vi "Show Detail.vi"(6 "mnu file Path 2":path, 7 "mnu file Path 1":path, 8 "error in (no error)":errorcluster, 9 "Palettes Different?":bool, 10 "Palette data array 2":T5(array[cluster]) {"view format" items=["Icons", "Text", "Icons and Text"]}, 11 "Palette data array 1":T5(array[cluster]) {"view format" items=["Icons", "Text", "Icons and Text"]}) -> (0 "error out":errorcluster)   [LabVIEW 2017]
uses:
  <vilib>/Palette API/Palette Menu/Public Type Define/View Format.ctl
  <vilib>/Palette API/Palette Menu/Public Type Define/Items.ctl
  <vilib>/Palette API/Palette Menu/Public Type Define/Item.ctl
  <vilib>/Palette API/Palette Menu/Public Type Define/Synchronize Info.ctl
  <vilib>/Palette API/Palette Menu/Palette Menu.lvlib
panel:
  out "Picture 2":picture
  in  "mnu file 2":string
  out "Picture 1":picture
  in  "mnu file 1":string
  in  "Palette information":string(tree)
  in  "View Format":T1 items=["Icons", "Text", "Icons and Text"]
  in  "stop":bool
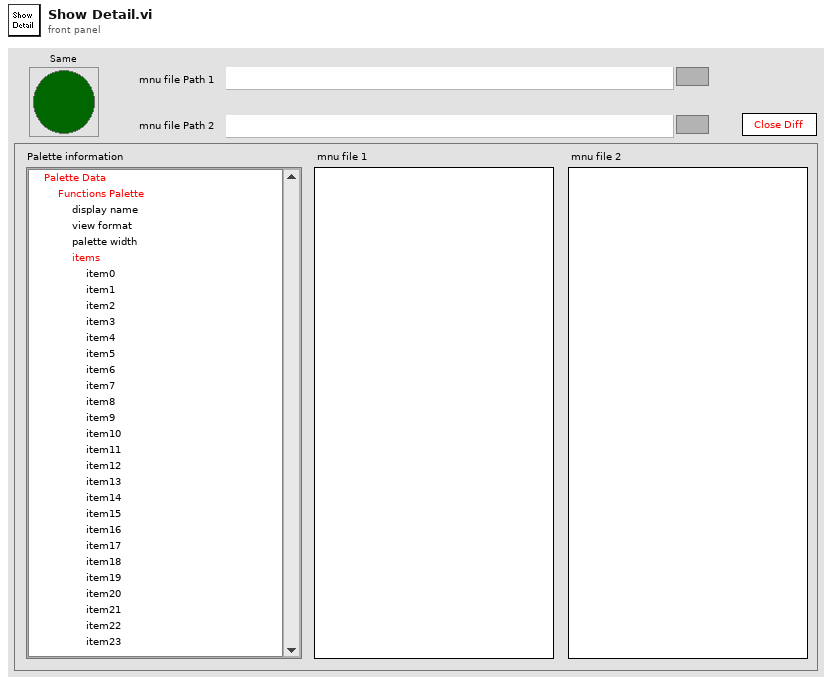
[diagram p1: front panel]
types:
  T1 = typedef "Palette Menu.lvlib/View Format.ctl" = u16
  T2 = typedef "Palette Menu.lvlib/Items.ctl" = T3[]
  T3 = typedef "Palette Menu.lvlib/Item.ctl" = cluster{"item path":path, "library path (.lvlib)":path, "use default lvlib palette":bool, "short name":string, "place VI contents":bool, "hide synchronized item":bool, "reserve spot for synch item":bool, "configure when placing VI contents":bool}
  T4 = typedef "Palette Menu.lvlib/Synchronize Info.ctl" = cluster{"synchronize with directory":bool, "synchronize directory path":path}
  T5 = cluster{"display name":string, "view format":T1, "palette width":i16, "items":T2, "256 color icon":picture, "B&W color icon":picture, "help information":cluster{"help tag":string, "help file path":path}, "palette description":string, "synchronize information":T4}[]
  T6 = enum32{"Invalid", "Standard", "Closed", "Hidden", "Minimized", "Maximized"}
  T7 = cluster{"display name":string, "view format":T1, "palette width":i16, "items":T2, "256 color icon":picture, "B&W color icon":picture, "help information":cluster{"help tag":string, "help file path":path}, "palette description":string, "synchronize information":T4}
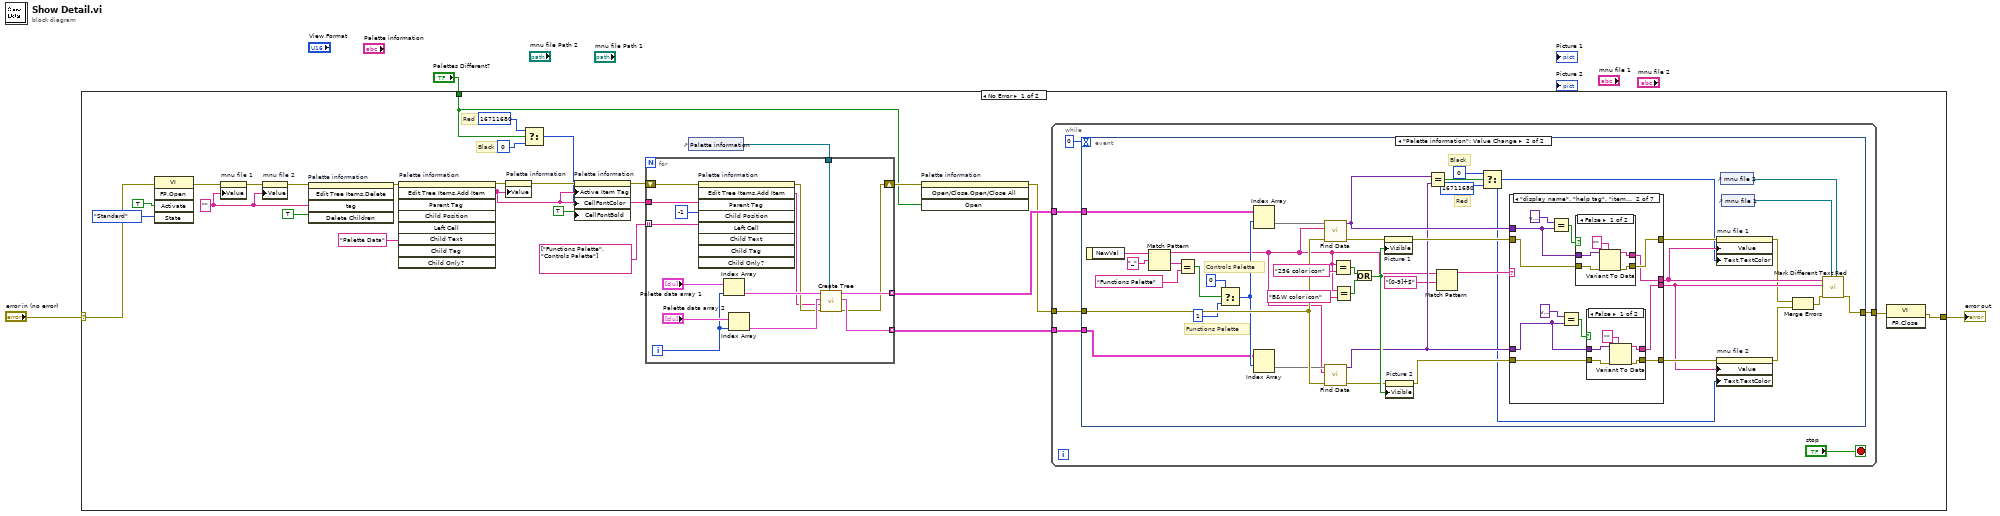
[diagram p0: block diagram]
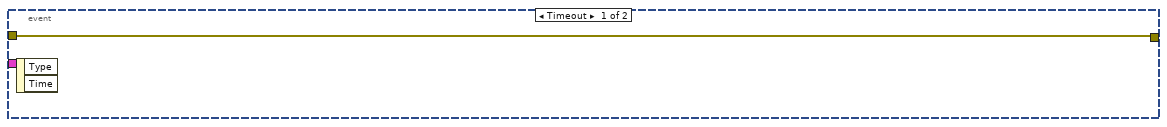
[diagram p2: hidden frame]
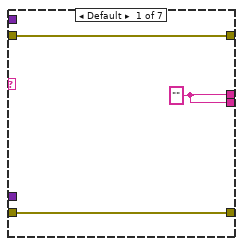
[diagram p3: hidden frame]
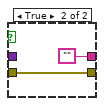
[diagram p4: hidden frame]
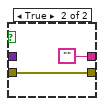
[diagram p5: hidden frame]
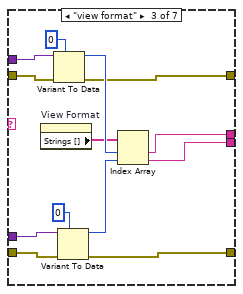
[diagram p6: hidden frame]
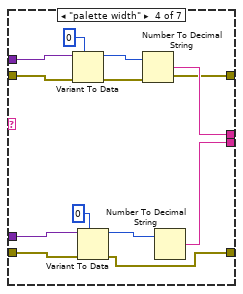
[diagram p7: hidden frame]
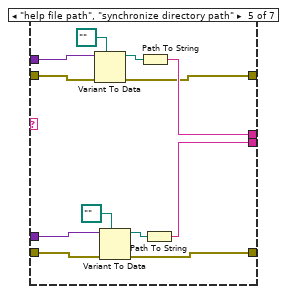
[diagram p8: hidden frame]
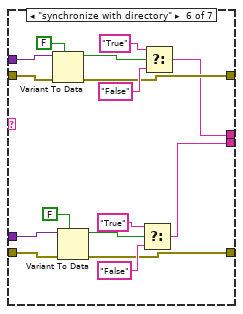
[diagram p9: hidden frame]
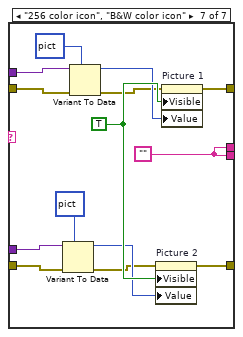
[diagram p10: hidden frame]
diagram:
  n1 = case shown="No Error" "error in (no error)" {
    selector: "error in (no error)" -> [w30 w190]
    tunnel: [w27 w190] -> w2
    tunnel: "Palettes Different?" -> [w4 _]
    frame No Error {
      w19 = "" ("Tag")
      # "Red"
      # "Black"
      n2 = invoke class="VI" method="FP.Open"(error in=w30, "Activate"=TRUE ("Activate?"), "State"=T6."Standard") -> (error out=w20:errorcluster)  [unwired: 2 in, 4 out]
      n3 = property on="mnu file 1" class="Str"(error in=w20, "Value"=w19) -> (error out=w22:errorcluster)  [unwired: 1 in, 1 out]
      n4 = property on="mnu file 2" class="Str"(error in=w22, "Value"=w19) -> (error out=w21:errorcluster)  [unwired: 1 in, 1 out]
      n5 = invoke on="Palette information" class="Tree (strict)" method="Edit Tree Items.Delete"(error in=w21, "tag"=w19, "Delete Children"=TRUE ("Delete Children?")) -> (error out=w25:errorcluster)  [unwired: 2 in, 4 out]
      n6 = invoke on="Palette information" class="Tree (strict)" method="Edit Tree Items.Add Item"(error in=w25, "Left Cell"="Palette Data" ("Left Cell String")) -> (error out=w18:errorcluster, "Edit Tree Items:Add Item"=w10:string)  [unwired: 7 in, 7 out]
      n7 = property on="Palette information" class="Tree (strict)"(error in=w18, "Value"=w10) -> (error out=w13:errorcluster)  [unwired: 1 in, 1 out]
      n8 = Select(t=u32 16711680, s=w4, f=u32 0 ("t")) -> (s? t:f=w9:u32)
      n9 = property on="Palette information" class="Tree (strict)"(error in=w13, "Active Item Tag"=w10, "CellFontColor"=w9, "CellFontBold"=TRUE ("Active Cell:Cell Font:Bold")) -> (error out=w7:errorcluster)  [unwired: 1 in, 1 out]
      n10 = control-ref of="Palette information"() -> (w16:refnum<vi>)
      n11 = for {
        tunnel: w10 -> [w44]
        tunnel: string[] ["Functions Palette", "Controls Palette"] ("Palette type") -> [w37] mode=indexing
        tunnel: w16 -> [w38]
        tunnel: [w35] -> w15 mode=indexing
        shift-right: [w31] -> w6
        shift-left: w7 -> [w34]
        tunnel: [w33] -> w14 mode=indexing
        i -> [w40]
        n12 = invoke on="Palette information" class="Tree (strict)" method="Edit Tree Items.Add Item"(error in=w34, "Parent Tag"=w44, "Child Position"=-1, "Left Cell"=w37) -> (error out=w36:errorcluster, "Edit Tree Items:Add Item"=w32:string)  [unwired: 5 in, 7 out]
        n13 = Index Array(array="Palette data array 1", index=w40) -> (element=w42:T7)
        n14 = Index Array(array="Palette data array 2", index=w40) -> (element=w39:T7)
        n15 = call "Create Tree.vi"("Tree Refnum"=w38, "error in"=w36, "Parent Tag"=w32, "palette data 2"=w39, "palette data 1"=w42) -> ("error out"=w31:errorcluster, "data array 2"=w33:cluster{"Label":string, "Data":variant}[], "data array 1"=w35:cluster{"Label":string, "Data":variant}[])  [unwired: 4 out]
      }
      n16 = invoke on="Palette information" class="Tree (strict)" method="Open/Close.Open/Close All"(error in=w6, "Open"=w4) -> (error out=w5:errorcluster)  [unwired: 2 in, 3 out]
      n17 = while {
        tunnel: w5 -> [w49]
        tunnel: [w48] -> w23
        tunnel: w15 -> [w47]
        tunnel: w14 -> [w46]
        stop <- "stop" stop-if-true
        n18 = event shown="[1] \"Palette information\": Value Change" {
          selector: _ -> [_ _]
          dyn-events: _ -> [_ _]
          timeout: 0 -> [_ _]
          tunnel: w49 -> [w52 w82]
          tunnel: [w52 w53] -> w48
          tunnel: w47 -> [_ w76]
          tunnel: w46 -> [_ w69]
          event Timeout {
            n19 = event-data() -> ()  [unwired: 3 out]
          }
          event "Palette information": Value Change {
            # "Controls Palette"
            # "Functions Palette"
            # "Red"
            # "Black"
            n20 = event-data() -> ("NewVal"=w73:string)  [unwired: 1 out]
            n21 = Match Pattern(string=w73, regular expression="_" ("search string")) -> (before substring=w63:string, after substring=w72:string)  [unwired: 3 out]
            n22 = Equal?(x=w72, y="Functions Palette") -> (x = y?=w70:bool)
            n23 = Select(t=0 ("y"), s=w70, f=1 ("y")) -> (s? t:f=w75:i32)
            n24 = Index Array(array=w76, index (row)=w75) -> (element=w67:cluster{"Label":string, "Data":variant}[])  [unwired: 1 in]
            n25 = Index Array(array=w69, index (row)=w75) -> (element=w66:cluster{"Label":string, "Data":variant}[])  [unwired: 1 in]
            n26 = call "Find Data.vi"("error in (no error)"=w82, "Label"=w63, "data array 1"=w67) -> ("error out"=w83:errorcluster, "Value"=w68:variant)  [unwired: 7 out]
            n27 = call "Find Data.vi"("error in (no error)"=w82, "Label"=w63, "data array 1"=w66) -> ("error out"=w81:errorcluster, "Value"=w65:variant)  [unwired: 1 in, 6 out]
            n28 = Equal?(x=w63, y="256 color icon") -> (x = y?=w91:bool)
            n29 = Equal?(x=w63, y="B&W color icon") -> (x = y?=w90:bool)
            n30 = Or(x=w91, y=w90) -> (x .or. y?=w89:bool)
            n31 = property on="Picture 1" class="Pict"(error in=w83, "Visible"=w89) -> (error out=w88:errorcluster)  [unwired: 1 in, 1 out]
            n32 = property on="Picture 2" class="Pict"(error in=w81, "Visible"=w89) -> (error out=w87:errorcluster)  [unwired: 1 in, 1 out]
            n33 = Equal?(x=w68, y=w65) -> (x = y?=w86:bool)
            n34 = Match Pattern(string=w63, regular expression="[0-9]+$") -> (before substring=w62:string)  [unwired: 4 out]
            n35 = Select(t=u32 0, s=w86, f=u32 16711680) -> (s? t:f=w58:u32)
            n36 = case shown="\"display name\", \"help tag\", \"item\", \"palette description\"" w62 {
              tunnel: w87 -> [w94 w99 w127 w141 w153 w165 w181]
              tunnel: w88 -> [w95 w108 w129 w142 w154 w166 w183]
              tunnel: w68 -> [_ w103 w130 w143 w155 w167 w184]
              tunnel: w65 -> [_ w100 w128 w140 w152 w164 w182]
              tunnel: [w96 w106 w126 w139 w149 w162 w178] -> w59
              tunnel: [w95 w107 w125 w138 w148 w163 w176] -> w80
              tunnel: [w96 w97 w124 w137 w151 w160 w178] -> w57
              tunnel: [w94 w98 w123 w136 w150 w161 w177] -> w79
              frame Default {
                w96 = ""
              }
              frame "display name", "help tag", "item", "palette description" {
                n37 = Equal?(x=variant ("y"), y=w103) -> (x = y?=w104:bool)
                n38 = Equal?(x=variant ("y"), y=w100) -> (x = y?=w101:bool)
                n39 = case shown="False" w104 {
                  tunnel: w108 -> [w119 w121]
                  tunnel: [w118 w121] -> w107
                  tunnel: [w117 ""] -> w106
                  tunnel: w103 -> [w116 _]
                  frame False {
                    n40 = Variant To Data(error in=w119, type="", Variant=w116) -> (data=w117:string, error out=w118:errorcluster)
                  }
                  frame True {
                  }
                }
                n41 = case shown="False" w101 {
                  tunnel: w99 -> [w112 w114]
                  tunnel: [w111 w114] -> w98
                  tunnel: [w110 ""] -> w97
                  tunnel: w100 -> [w109 _]
                  frame False {
                    n42 = Variant To Data(error in=w112, type="", Variant=w109) -> (data=w110:string, error out=w111:errorcluster)
                  }
                  frame True {
                  }
                }
              }
              frame "view format" {
                n43 = property on="View Format" class="Ring (strict)"() -> ("Strings []"=w133:string[])  [unwired: 2 in, 2 out]
                n44 = Variant To Data(error in=w129, type=0, Variant=w130) -> (data=w134:i32, error out=w125:errorcluster)
                n45 = Variant To Data(error in=w127, type=0, Variant=w128) -> (data=w131:i32, error out=w123:errorcluster)
                n46 = Index Array(array=w133, index #1=w134, index #2=w131) -> (element #1=w126:string, element #2=w124:string)
              }
              frame "palette width" {
                n47 = Variant To Data(error in=w142, type=0, Variant=w143) -> (data=w147:i32, error out=w138:errorcluster)
                n48 = Variant To Data(error in=w141, type=0, Variant=w140) -> (data=w146:i32, error out=w136:errorcluster)
                n49 = Number To Decimal String(number=w147) -> (decimal integer string=w139:string)  [unwired: 1 out]
                n50 = Number To Decimal String(number=w146) -> (decimal integer string=w137:string)  [unwired: 1 out]
              }
              frame "help file path", "synchronize directory path" {
                n51 = Variant To Data(error in=w154, type=path "", Variant=w155) -> (data=w157:path, error out=w148:errorcluster)
                n52 = Variant To Data(error in=w153, type=path "", Variant=w152) -> (data=w156:path, error out=w150:errorcluster)
                n53 = Path To String(path=w157) -> (string=w149:string)
                n54 = Path To String(path=w156) -> (string=w151:string)
              }
              frame "synchronize with directory" {
                n55 = Variant To Data(error in=w166, type=FALSE, Variant=w167) -> (data=w168:bool, error out=w163:errorcluster)
                n56 = Variant To Data(error in=w165, type=FALSE, Variant=w164) -> (data=w174:bool, error out=w161:errorcluster)
                n57 = Select(t="True", s=w174, f="False") -> (s? t:f=w160:string)
                n58 = Select(t="True", s=w168, f="False") -> (s? t:f=w162:string)
              }
              frame "256 color icon", "B&W color icon" {
                w189 = TRUE
                w178 = ""
                n59 = Variant To Data(error in=w181, type=picture data[5B] ("Picture 1"), Variant=w182) -> (data=w185:picture, error out=w179:errorcluster)
                n60 = Variant To Data(error in=w183, type=picture data[5B] ("Picture 1"), Variant=w184) -> (data=w187:picture, error out=w180:errorcluster)
                n61 = property on="Picture 2" class="Pict"(error in=w179, "Visible"=w189, "Value"=w185) -> (error out=w177:errorcluster)  [unwired: 1 in, 1 out]
                n62 = property on="Picture 1" class="Pict"(error in=w180, "Visible"=w189, "Value"=w187) -> (error out=w176:errorcluster)  [unwired: 1 in, 1 out]
              }
            }
            n63 = property on="mnu file 1" class="Str"(error in=w80, "Value"=w59, "Text.TextColor"=w58) -> (error out=w55:errorcluster)  [unwired: 1 in, 1 out]
            n64 = property on="mnu file 2" class="Str"(error in=w79, "Value"=w57, "Text.TextColor"=w58) -> (error out=w56:errorcluster)  [unwired: 1 in, 1 out]
            n65 = control-ref of="mnu file 2"() -> (w60:refnum<vi>)
            n66 = control-ref of="mnu file 1"() -> (w61:refnum<vi>)
            n67 = Merge Errors(w55, w56) -> (w54:errorcluster)
            n68 = call "Mark Different Text Red.vi"("reference 2"=w60, "reference 1"=w61, "error in (no error)"=w54, "String 2"=w57, "String1"=w59) -> ("error out"=w53:errorcluster)  [unwired: 6 out]
          }
        }
      }
      n69 = invoke class="VI" method="FP.Close"(error in=w23) -> (error out=w27:errorcluster)  [unwired: 2 in, 2 out]
    }
    frame Error {
    }
  }
  "error out" <- w2
